vi "Connection Close.vi"(8 "error in (no error)":errorcluster, 11 "VISA resource name In":T1={"Conection Data"="COM4"}) -> (0 "error out":errorcluster, 3 "VISA resource name Out":T1={"Conection Data"="COM4"})   [LabVIEW 2014, in "AD4212C Lib.lvlib"]
doc: "Cierra el puerto COM de la pc."
uses:
  AD4212C Lib.lvlib
  Typedef/Connection Data.ctl
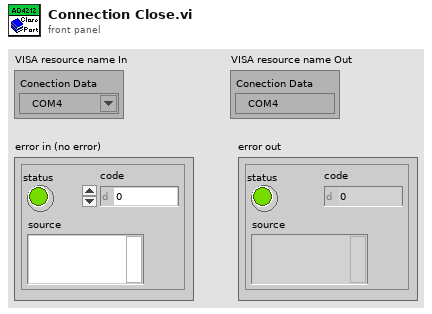
[diagram p1: front panel]
types:
  T1 = typedef "AD4212C Lib.lvlib/Connection Data.ctl" = cluster{"Conection Data":refnum<visa-resource-name>}
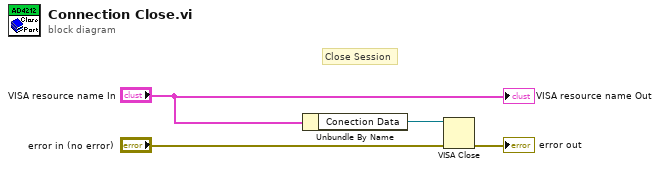
[diagram p0: block diagram]
diagram:
  # "Close Session"
  n1 = Unbundle By Name("VISA resource name In") -> ("Conection Data"=w2:refnum<visa-resource-name>)
  n2 = VISA Close(VISA resource name=w2, error in (no error)="error in (no error)") -> (error out=→"error out":errorcluster)
  "VISA resource name Out" <- "VISA resource name In"
